vi "Get Info.vi"(8 "error in (no error)":errorcluster, 11 "Statement in":refnum<class "Statement.lvclass">) -> (0 "error out":errorcluster, 1 "Transaction Count":i32, 2 "First Transaction":refnum<class "Transaction.lvclass">, 3 "Statement out":refnum<class "Statement.lvclass">)   [LabVIEW 2018, in "Statement.lvclass"]
uses:
  Statement.lvclass
  Transaction/Transaction.lvclass
  Statement.lvclass/Statement.ctl
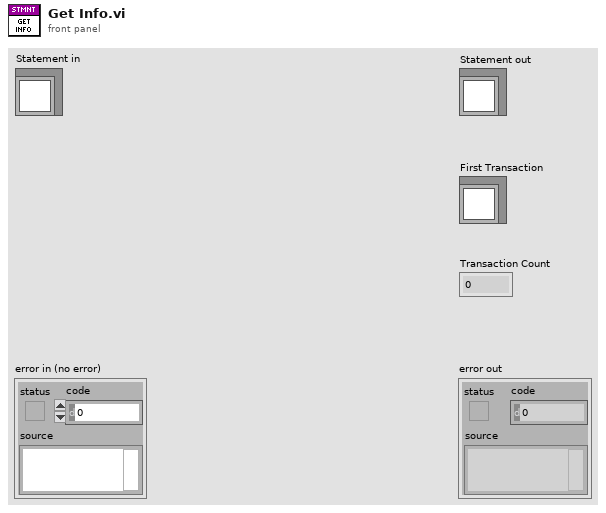
[diagram p1: front panel]
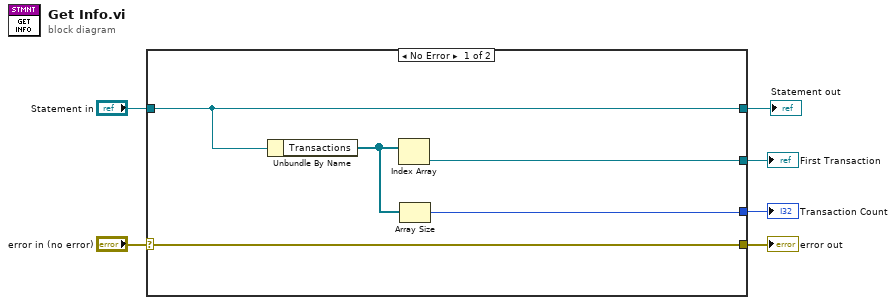
[diagram p0: block diagram]
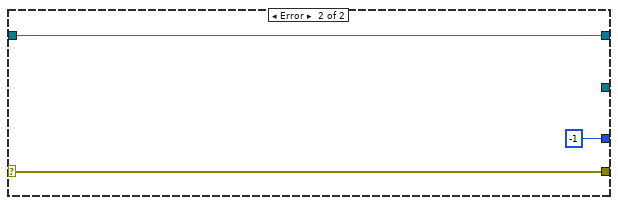
[diagram p2: hidden frame]
diagram:
  n1 = case shown="No Error" "error in (no error)" {
    selector: "error in (no error)" -> [w11 w14]
    tunnel: [w11 w14] -> w5
    tunnel: "Statement in" -> [w7 w12]
    tunnel: [w10 _] -> w3
    tunnel: [w8 -1] -> w2
    tunnel: [w7 w12] -> w1
    frame No Error {
      n2 = Unbundle By Name(w7) -> ("Transactions"=w9:refnum<class "Transaction.lvclass">[])
      n3 = Index Array(array=w9) -> (element=w10:refnum<class "Transaction.lvclass">)  [unwired: 1 in]
      n4 = Array Size(array=w9) -> (size(s)=w8:i32)
    }
    frame Error {
    }
  }
  "error out" <- w5
  "First Transaction" <- w3
  "Transaction Count" <- w2
  "Statement out" <- w1
